vi "DIConfigurationSubVI.vi"(8 "error in":errorcluster, 10 "Sim?":bool, 11 "Input Lines":tag) -> (0 "error out":errorcluster, 3 "task out":refnum<k21>)   [LabVIEW 2017]
uses:
  <vilib>/DAQmx/create/channels.llb/DAQmx Create Channel (DI-Digital Input).vi
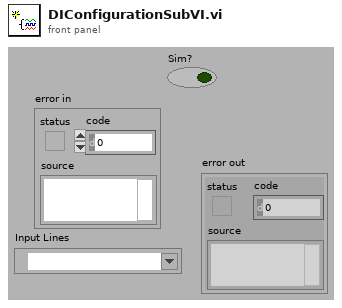
[diagram p1: front panel]
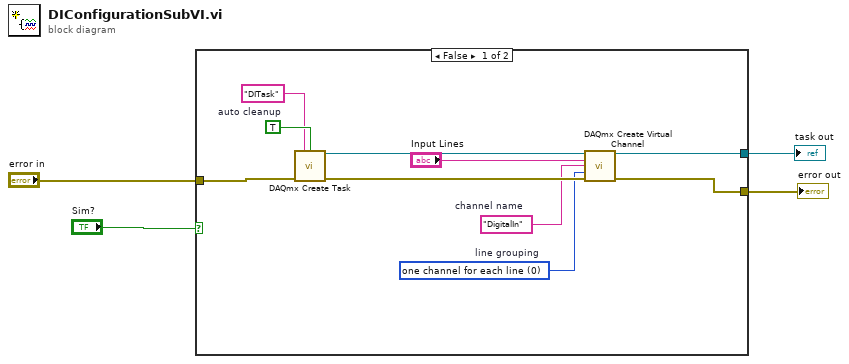
[diagram p0: block diagram]
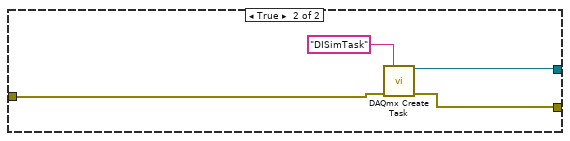
[diagram p2: hidden frame]
diagram:
  n1 = case shown="False" "Sim?" {
    tunnel: "error in" -> [w14 w15]
    tunnel: [w8 w17] -> w3
    tunnel: [w7 w16] -> w2
    frame False {
      w10 = 0 items=["one channel for each line", "one channel for all lines"]  # line grouping
      w9 = "DigitalIn"  # channel name
      w12 = TRUE  # auto cleanup
      n2 = call <vilib>:"DAQmx Create Task.vi"("new task name"="DITask", "auto cleanup"=w12, "error in"=w14) -> ("task out"=w11:refnum<k21>, "error out"=w13:errorcluster)  [unwired: 11 in]
      n3 = call-poly <vilib>:"DAQmx Create Virtual Channel.vi"("task in"=w11, "lines"="Input Lines", "name to assign"=w9, "line grouping"=w10, "error in"=w13) -> ("task out"=w8:refnum<k21>, "error out"=w7:errorcluster)  [unwired: 9 in]
    }
    frame True {
      n4 = call <vilib>:"DAQmx Create Task.vi"("new task name"="DISimTask", "error in"=w15) -> ("task out"=w17:refnum<k21>, "error out"=w16:errorcluster)  [unwired: 12 in]
    }
  }
  "error out" <- w2
  "task out" <- w3
